vi "Resource.vi"(6 "action":enum16{"Get", "Lock", "unlock"}(ring), 8 "error in (no error)":errorcluster, 11 "input":variant) -> (0 "error out":errorcluster, 2 "Queue out":refnum<queue>, 3 "GlobalCacher":variant)   [LabVIEW 2017, in "ObjectCacherAPI.lvlib"]
uses:
  ObjectCacherAPI.lvlib
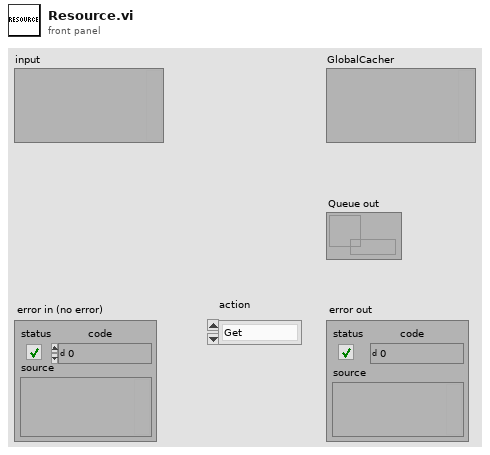
[diagram p1: front panel]
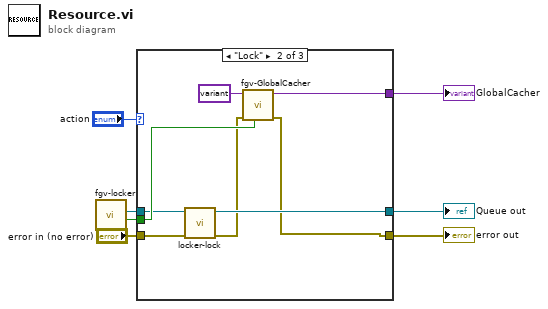
[diagram p0: block diagram]
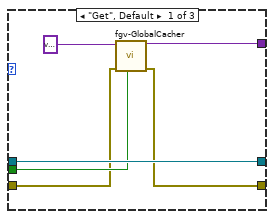
[diagram p2: hidden frame]
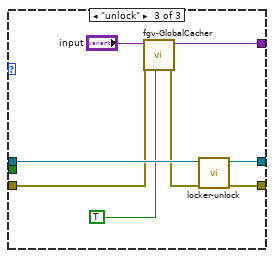
[diagram p3: hidden frame]
diagram:
  n1 = call "fgv-locker.vi"() -> ("create new?"=w1:bool, "Queue out"=w2:refnum<queue>)  [unwired: 10 in]
  n2 = case shown="\"Lock\"" "action" {
    tunnel: [w11 w20 w24] -> w7
    tunnel: [w13 w21 w29] -> w5
    tunnel: [w8 w14 w28] -> w4
    tunnel: "error in (no error)" -> [w9 w17 w22]
    tunnel: w2 -> [w13 w16 w27]
    tunnel: w1 -> [w10 w18 _]
    frame "Get", Default {
      n3 = call "fgv-GlobalCacher.vi"("Boolean"=w10, "error in (no error)"=w9, "Variant (in)"=variant) -> ("error out"=w8:errorcluster, "Variant"=w11:variant)  [unwired: 7 in]
    }
    frame "Lock" {
      n4 = call "locker-lock.vi"("error in (no error)"=w17, "queue"=w16) -> ("error out"=w15:errorcluster, "Queue out"=w21:refnum<queue>)  [unwired: 8 in]
      n5 = call "fgv-GlobalCacher.vi"("Boolean"=w18, "error in (no error)"=w15, "Variant (in)"=variant) -> ("error out"=w14:errorcluster, "Variant"=w20:variant)  [unwired: 7 in]
    }
    frame "unlock" {
      n6 = call "fgv-GlobalCacher.vi"("Boolean"=TRUE, "error in (no error)"=w22, "Variant (in)"="input") -> ("error out"=w23:errorcluster, "Variant"=w24:variant)  [unwired: 7 in]
      n7 = call "locker-unlock.vi"("error in (no error)"=w23, "Queue in"=w27) -> ("error out"=w28:errorcluster, "Queue out"=w29:refnum<queue>)  [unwired: 8 in]
    }
  }
  "GlobalCacher" <- w7
  "error out" <- w4
  "Queue out" <- w5
